vi "DeletePoint.vi"(8 "error in":errorcluster, 10 "Cluster in":T3={"Calibration Input"=[], "CalibrationResults"={"Center in Pixels"=[374.0120339529387, 375.46592887074246], "Angle"=0.022945275255000355, "Pixels/MHz X"=0.0, "Pixels/MHz Y"=0.0}, "Highlight"=[], "Running Script"=refnum}, 11 "Queues Input":T1) -> (0 "error out":errorcluster)   [LabVIEW 2017]
uses:
  TypeDefinitions/ExperimentVariables.ctl
  TypeDefinitions/SubVIQueues.ctl
  AODControl/MessageQueue/QueueOperations/All Message Queues.ctl
  AODControl/MessageQueue/QueueOperations/Message Cluster.ctl
  AODControl/AODControlFiles/AODPointDefinition.ctl
  MessageQueue/QueueOperations/Enqueue Message (Single).vi
  MessageQueue/MessageQueue.lvlib
  AODControl/AODControl.lvlib
  AODControl/MessageQueue/MessageQueue.lvlib
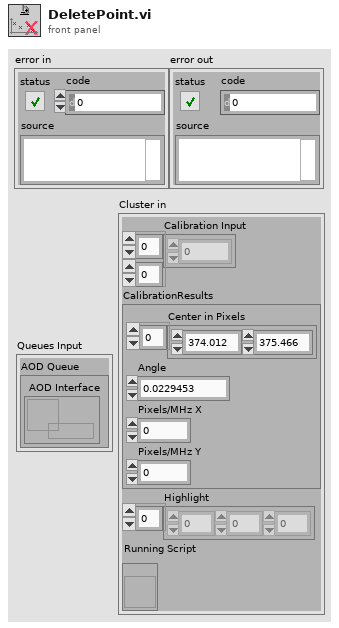
[diagram p1: front panel]
types:
  T1 = typedef "SubVIQueues.ctl" = cluster{"AOD Queue":T2}
  T2 = typedef "AODControl.lvlib/MessageQueue.lvlib/All Message Queues.ctl" = cluster{" AOD Interface":refnum<queue>}
  T3 = typedef "ExperimentVariables.ctl" = cluster{"Calibration Input":i32[][], "CalibrationResults":cluster{"Center in Pixels":dbl[], "Angle":dbl, "Pixels/MHz X":dbl, "Pixels/MHz Y":dbl}, "Highlight":i32[], "Running Script":refnum<vi>}
  T4 = typedef "AODControl.lvlib/AODPointDefinition.ctl" = cluster{"Freq X":dbl, "Freq Y":dbl, "Index":i32, "Ampitude":dbl}
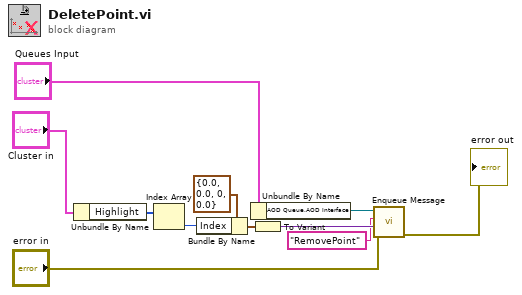
[diagram p0: block diagram]
diagram:
  n1 = Unbundle By Name("Cluster in") -> ("Highlight"=w5:i32[])
  n2 = Index Array(array=w5) -> (element=w9:i32)  [unwired: 1 in]
  n3 = Bundle By Name(cluster=T4 {"Freq X"=0.0, "Freq Y"=0.0, "Index"=0, "Ampitude"=0.0} ("Cluster"), "Index"=w9) -> (w10:T4)
  n4 = Unbundle By Name("Queues Input") -> ("AOD Queue.AOD Interface"=w3:refnum<queue>)
  n5 = To Variant(anything=w10) -> (Variant=w6:variant)
  n6 = call-poly "Enqueue Message.vi"("error in (no error)"="error in", "Message Data"=w6, "Message"="RemovePoint", "Message Queue"=w3) -> ("error out"=→"error out":errorcluster)  [unwired: 6 in, 1 out]
